vi "niRFUtil WFM Remove Quadrature Error - Coarse.vi"(0 "Descrambled Chips In":T1 {"y" format="%.2f"; "dx" format="%^.2e"; "x0" format="%^.2e"}) -> (2 "Corrected Descrambled Chips Out":T1 {"y" format="%.2f"; "dx" format="%^.2e"; "x0" format="%^.2e"}, 3 "Phase Imbalance (deg)":sgl format="%.4f")   [LabVIEW 2015, in "niRFUtil.lvlib"]
doc: "(c) Copyright 2006, National Instruments, Inc. This VI may not be duplicated, sold, or distributed without written consent from National Instruments."
uses:
  niRFUtil.lvlib
  Includes/niRFUtil INC Complex Waveform.ctl
  Includes/niRFUtil INC Complex Array.ctl
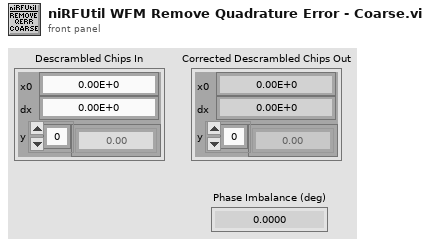
[diagram p1: front panel]
types:
  T1 = typedef "niRFUtil.lvlib/niRFUtil INC Complex Waveform.ctl" = cluster{"x0":dbl, "dx":dbl, "y":T2}
  T2 = typedef "niRFUtil.lvlib/niRFUtil INC Complex Array.ctl" = csg[]
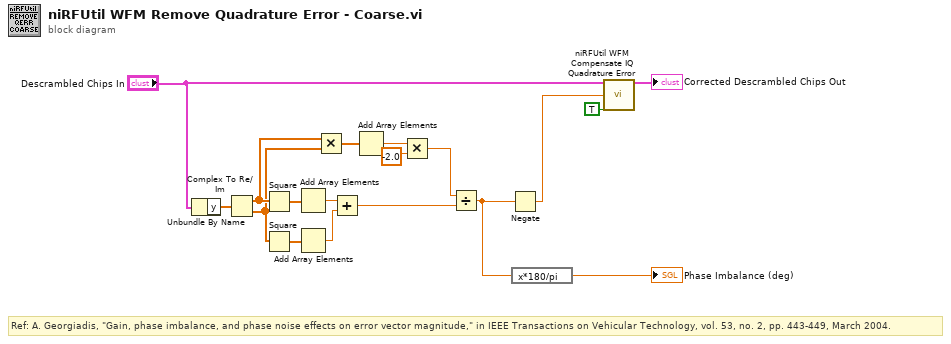
[diagram p0: block diagram]
diagram:
  # "Ref: A. Georgiadis, \"Gain, phase imbalance, and phase noise effects on error vector magnitude,\" in IEEE Transactions on Vehicular Technology, vol. 53, no. 2, pp. 443-449, March 2004."
  n1 = Unbundle By Name("Descrambled Chips In") -> ("y"=w18:T2)
  n2 = Complex To Re/Im(x + iy=w18) -> (x=w11:sgl[], y=w10:sgl[])
  n3 = Square(x=w11) -> (x^2=w17:sgl[])
  n4 = Square(x=w10) -> (x^2=w16:sgl[])
  n5 = Add Array Elements(numeric array=w17) -> (sum=w15:sgl)
  n6 = Add Array Elements(numeric array=w16) -> (sum=w14:sgl)
  n7 = Multiply(x=w11, y=w10) -> (x*y=w9:sgl[])
  n8 = Add(x=w15, y=w14) -> (x+y=w6:sgl)
  n9 = Add Array Elements(numeric array=w9) -> (sum=w8:sgl)
  n10 = Multiply(x=w8, y=sgl -2.0) -> (x*y=w5:sgl)
  n11 = Divide(x=w5, y=w6) -> (x/y=w1:sgl)
  n12 = Negate(x=w1) -> (-x=w3:sgl)
  n13 = expression code="x*180/pi"(w1) -> (→"Phase Imbalance (deg)":sgl)
  n14 = call "niRFUtil WFM Compensate IQ Quadrature Error.vi"("Input"="Descrambled Chips In", "Phase Imbalance (rad)"=w3, "Compensate?"=TRUE) -> ("Waveform Out"=→"Corrected Descrambled Chips Out":T1)  [unwired: 12 in]
